vi "ReadStatus.vi"(8 "error in (no error)":errorcluster, 10 "XPath expression":string="/COOLER_STATUS/LIST_OF_PROPERTIES/PROPERTY", 11 "path to XML document":path caption="path to XML") -> (0 "error out":errorcluster, 1 "value":string[](array[string]), 2 "units":string[](array[string]), 3 "Properties":string[](array[string]))   [LabVIEW 2017]
uses:
  <vilib>/xml/Load XML File.vi
  <vilib>/xml/Close Reference(Node).vi
  <vilib>/xml/NI_XML.lvlib
  <resource>/objmgr/DOMUserDefRef.rc
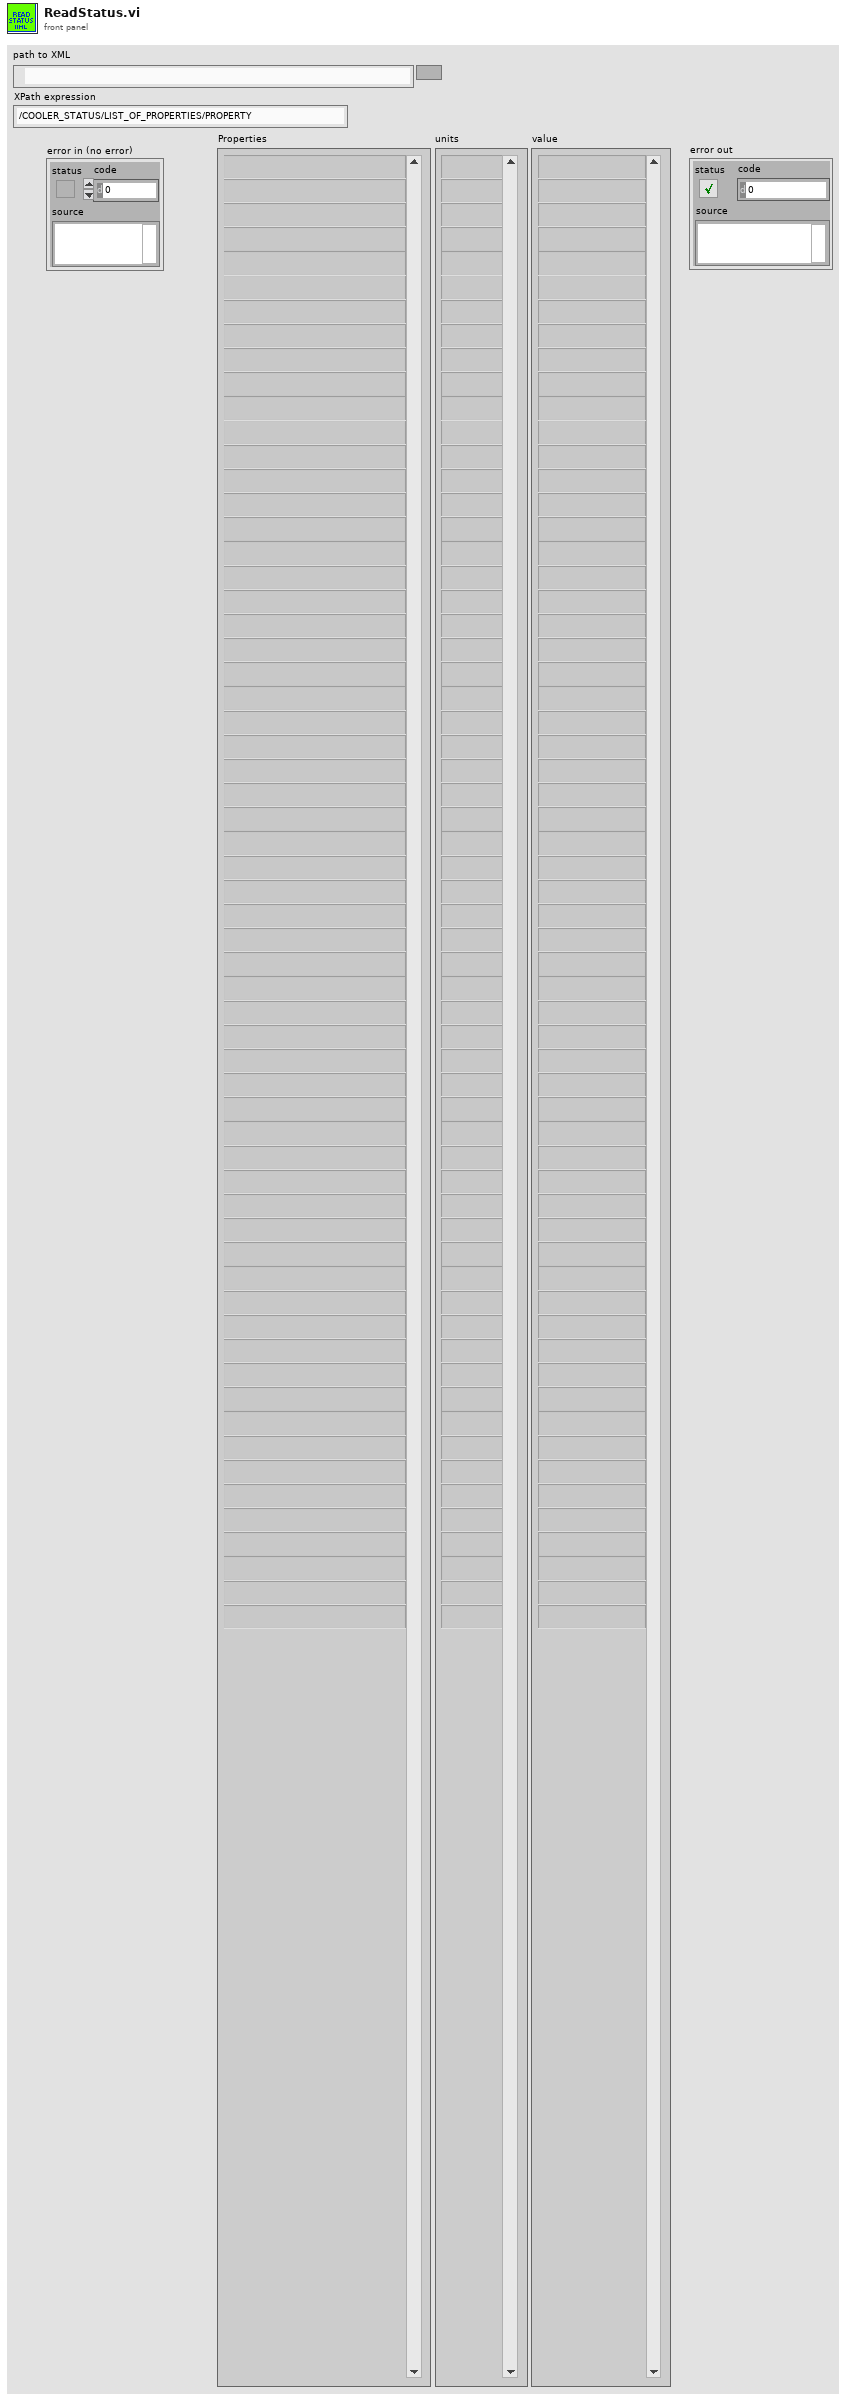
[diagram p1: front panel]
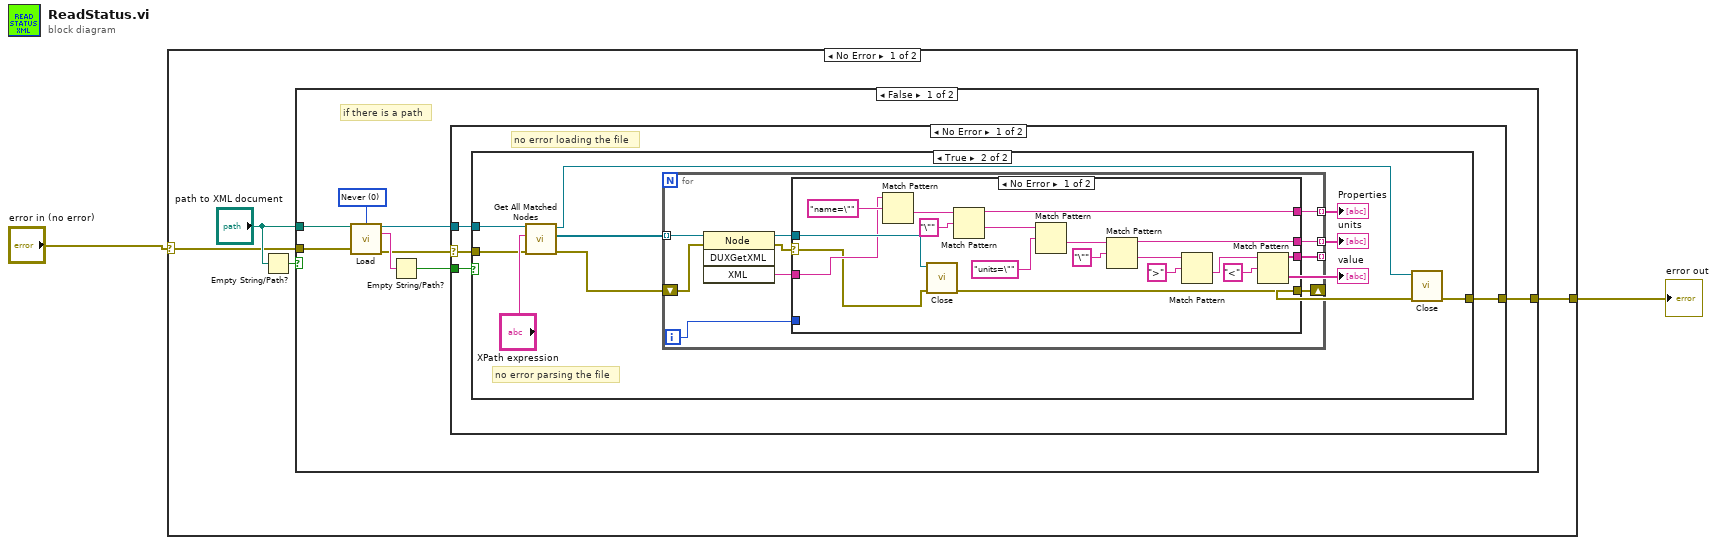
[diagram p0: block diagram]
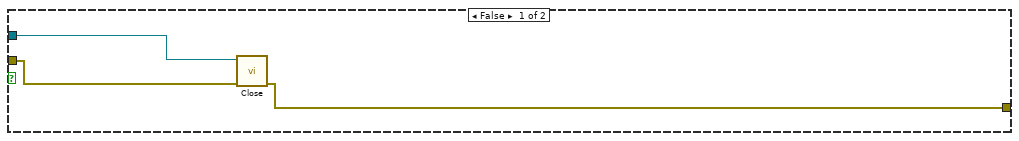
[diagram p2: hidden frame]
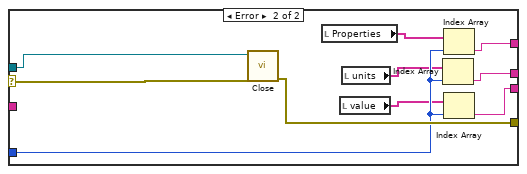
[diagram p3: hidden frame]
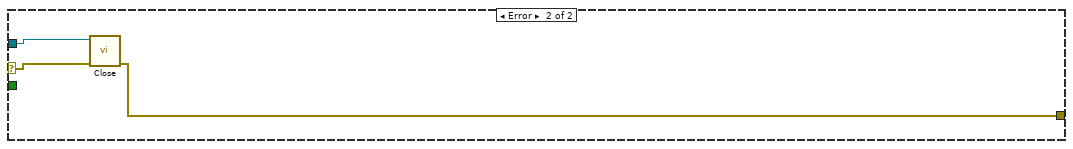
[diagram p4: hidden frame]
diagram:
  n1 = case shown="No Error" "error in (no error)" {
    selector: "error in (no error)" -> [w3 w75]
    tunnel: [w4 w75] -> w2
    frame No Error {
      n2 = Empty String/Path?(string/path="path to XML document") -> (empty?=w6:bool)
      n3 = case shown="False" w6 {
        tunnel: "path to XML document" -> [w13 _]
        tunnel: w3 -> [w12 w74]
        tunnel: [w11 w74] -> w4
        frame False {
          w7 = 0 items=["Never", "Always", "Auto"] ("validate on load (Auto)")
          # "if there is a path"
          n4 = call-poly <vilib>:"Load.vi"("path to XML document"=w13, "validate on load (Auto)"=w7, "error in (no error)"=w12) -> ("DOM document out"=w14:refnum<k20>, "parse errors"=w10:string, "error out"=w8:errorcluster)  [unwired: 10 in]
          n5 = Empty String/Path?(string/path=w10) -> (empty?=w9:bool)
          n6 = case shown="No Error" w8 {
            selector: w8 -> [w15 w73]
            tunnel: w14 -> [w18 w71]
            tunnel: [w17 w72] -> w11
            tunnel: w9 -> [w16 _]
            frame No Error {
              # "no error loading the file"
              n7 = case shown="True" w16 {
                tunnel: w18 -> [w20 w32]
                tunnel: [w21 w24] -> w17
                tunnel: w15 -> [w19 w22]
                frame False {
                  n8 = call-poly <vilib>:"Close.vi"("error in (no error)"=w19, "node"=w20) -> ("error out"=w21:errorcluster)  [unwired: 7 in]
                }
                frame True {
                  # "no error parsing the file"
                  n9 = call <vilib>:"Get All Matched Nodes.vi"("error in (no error)"=w22, "XPath expression"="XPath expression", "node in"=w32) -> ("error out"=w23:errorcluster, "node result array"=w31:refnum<k20>[], "node out"=w26:refnum<k20>)  [unwired: 6 out]
                  n10 = for {
                    tunnel: w31 -> [w37] mode=indexing
                    tunnel: [w42] -> w29 mode=indexing
                    tunnel: [w41] -> w28 mode=indexing
                    tunnel: [w40] -> w30 mode=indexing
                    shift-right: [w39] -> w25
                    shift-left: w23 -> [w38]
                    i -> [w33]
                    n11 = invoke class="Node" method="DUXGetXML"(reference=w37, error in=w38) -> (reference out=w36:refnum<k20>, error out=w34:errorcluster, "XML"=w35:string)  [unwired: 2 in, 1 out]
                    n12 = case shown="No Error" w34 {
                      selector: w34 -> [w43 w61]
                      tunnel: [w49 w67] -> w42
                      tunnel: [w48 w63] -> w41
                      tunnel: [w47 w62] -> w40
                      tunnel: [w46 w70] -> w39
                      tunnel: w36 -> [w45 w69]
                      tunnel: w35 -> [w44 _]
                      tunnel: w33 -> [_ w66]
                      frame No Error {
                        n13 = Match Pattern(string=w44, regular expression="name=\"") -> (after substring=w59:string)  [unwired: 1 in, 3 out]
                        n14 = call-poly <vilib>:"Close.vi"("error in (no error)"=w43, "node"=w45) -> ("error out"=w46:errorcluster)  [unwired: 7 out]
                        n15 = Match Pattern(string=w59, regular expression="\"") -> (before substring=w49:string, after substring=w54:string)  [unwired: 1 in, 2 out]
                        n16 = Match Pattern(string=w54, regular expression="units=\"") -> (after substring=w56:string)  [unwired: 1 in, 3 out]
                        n17 = Match Pattern(string=w56, regular expression="\"") -> (before substring=w48:string, after substring=w50:string)  [unwired: 1 in, 2 out]
                        n18 = Match Pattern(string=w50, regular expression=">") -> (after substring=w52:string)  [unwired: 1 in, 3 out]
                        n19 = Match Pattern(string=w52, regular expression="<") -> (before substring=w47:string)  [unwired: 1 in, 3 out]
                      }
                      frame Error {
                        n20 = call-poly <vilib>:"Close.vi"("error in (no error)"=w61, "node"=w69) -> ("error out"=w70:errorcluster)  [unwired: 7 in]
                        n21 = local read "Properties"() -> (w68:string[])
                        n22 = local read "value"() -> (w64:string[])
                        n23 = local read "units"() -> (w65:string[])
                        n24 = Index Array(array=w65, index=w66) -> (element=w63:string)
                        n25 = Index Array(array=w68, index=w66) -> (element=w67:string)
                        n26 = Index Array(array=w64, index=w66) -> (element=w62:string)
                      }
                    }
                  }
                  "Properties" <- w29
                  "units" <- w28
                  "value" <- w30
                  n27 = call-poly <vilib>:"Close.vi"("error in (no error)"=w25, "node"=w26) -> ("error out"=w24:errorcluster)  [unwired: 7 out]
                }
              }
            }
            frame Error {
              n28 = call-poly <vilib>:"Close.vi"("error in (no error)"=w73, "node"=w71) -> ("error out"=w72:errorcluster)  [unwired: 7 in]
            }
          }
        }
        frame True {
          # "if there is a path"
        }
      }
    }
    frame Error {
    }
  }
  "error out" <- w2
